vi "DLE destuffing 19092022 (1).vi"(4 "DLE stuffed input":u8[](array[numeric])) -> (1 "DLE destuffed output":u8[](array[numeric]))   [LabVIEW 2021]
panel:
  # "DLE (16) Decoding is done when duplicate is present"
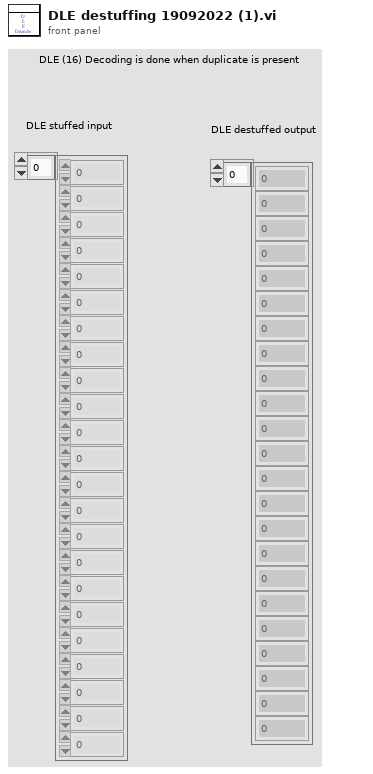
[diagram p1: front panel]
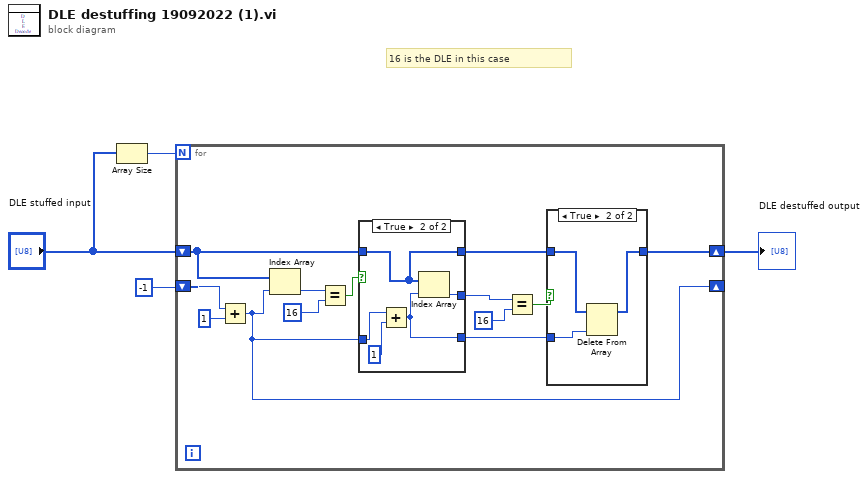
[diagram p0: block diagram]
diagram:
  # "16 is the DLE in this case"
  n1 = Array Size(array="DLE stuffed input") -> (size(s)=w1:i32)
  n2 = for {
    N: w1 -> [_]
    shift-right: [w13] -> _
    shift-left: -1 -> [w17]
    shift-right: [w8] -> w2
    shift-left: "DLE stuffed input" -> [w9]
    n3 = Add(x=w17, y=1) -> (x+y=w13:i32)
    n4 = Index Array(array=w9, index=w13) -> (element=w15:u8)
    n5 = Equal?(x=w15, y=u16 16) -> (x = y?=w14:bool)
    n6 = case shown="True" w14 {
      tunnel: w9 -> [w22 w23]
      tunnel: w13 -> [_ w27]
      tunnel: [w22 w23] -> w7
      tunnel: [_ w25] -> w12
      tunnel: [_ w24] -> w6
      frame False {
      }
      frame True {
        n7 = Add(x=w27, y=1) -> (x+y=w24:i32)
        n8 = Index Array(array=w23, index=w24) -> (element=w25:u8)
      }
    }
    n9 = Equal?(x=w12, y=u16 16) -> (x = y?=w10:bool)
    n10 = case shown="True" w10 {
      tunnel: w7 -> [w18 w21]
      tunnel: [w18 w20] -> w8
      tunnel: w6 -> [_ w19]
      frame False {
      }
      frame True {
        n11 = Delete From Array(array=w21, index=w19) -> (array with subset deleted=w20:u8[])  [unwired: 1 in, 1 out]
      }
    }
  }
  "DLE destuffed output" <- w2
